vi "WPI_DMARead.vi"(8 "error in (no error)":errorcluster, 9 "Timeout":dbl=5.0, 10 "SamplesToRead":u32=1, 11 "DMARef":T1) -> (0 "error out":errorcluster, 1 "Overrun":bool, 2 "Data":string, 3 "DMARef":T1, 4 "Samples Remaining":u32, 5 "Timed Out":bool)   [LabVIEW 2017]
doc: "Copies and returns the data out of the host buffer.\n\nThis software is licensed. Open the labview\\readme\\WPI Robotics Library Open Source License.txt file for more information."
uses:
  <vilib>/Rock Robotics/WPI/DMA/WPI_DMARef.ctl
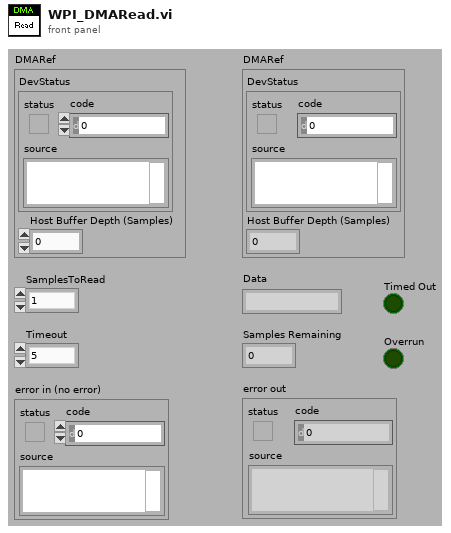
[diagram p1: front panel]
types:
  T1 = typedef "WPI_DMARef.ctl" = cluster{"DevStatus":errorcluster, "Host Buffer Depth (Samples)":u32}
  T2 = typedef "FPGA_DMADevRef.ctl" = cluster{"DevStatus":errorcluster}
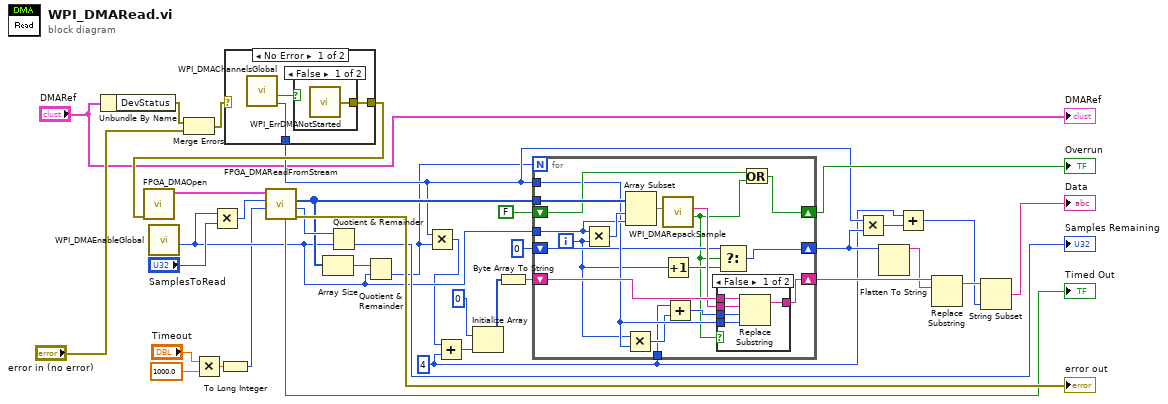
[diagram p0: block diagram]
diagram:
  w6 = u32 4 ("y")
  n1 = Unbundle By Name("DMARef") -> ("DevStatus"=w4:errorcluster)
  n2 = call <vilib>:"WPI_DMAEnableGlobal.vi"() -> ("WordsPerSample"=w21:u16)  [unwired: 2 in, 9 out]
  n3 = Merge Errors(w4, "error in (no error)") -> (w3:errorcluster)
  n4 = Multiply(x="Timeout", y=1000.0) -> (x*y=w29:dbl)
  n5 = Multiply(x=w21, y="SamplesToRead") -> (x*y=w27:u32)
  n6 = To Long Integer(number=w29) -> (32bit integer=w5:i32)
  n7 = case shown="No Error" w3 {
    selector: w3 -> [_ w42]
    tunnel: [w39 w42] -> w32
    tunnel: [w38 _] -> w14
    frame No Error {
      n8 = call <vilib>:"WPI_DMAChannelsGlobal.vi"() -> ("Packed Bytes Per Sample"=w38:i32, "Started"=w40:bool)  [unwired: 4 in, 6 out]
      n9 = case shown="False" w40 {
        tunnel: [w41 _] -> w39
        frame False {
          n10 = call <vilib>:"WPI_ErrDMANotStarted.vi"() -> ("error out"=w41:errorcluster)
        }
        frame True {
        }
      }
    }
    frame Error {
    }
  }
  n11 = call <vilib>:"FPGA_DMAOpen.vi"("error in (no error)"=w32) -> ("DMADevRef"=w28:T2)  [unwired: 10 out]
  n12 = call <vilib>:"FPGA_DMAReadFromStream.vi"("Timeout (ms)"=w5, "NumberOfElements"=w27, "DMADevRef In"=w28) -> ("error out"=→"error out":errorcluster, "Elements Remaining"=w25:u32, "Data"=w23:u32[], "Timed Out"=→"Timed Out":bool)  [unwired: 1 in, 4 out]
  n13 = Array Size(array=w23) -> (size(s)=w24:i32)
  n14 = Quotient & Remainder(x=w25, y=w21) -> (floor(x/y)=→"Samples Remaining":u32)  [unwired: 1 out]
  n15 = Quotient & Remainder(x=w24, y=w21) -> (floor(x/y)=w13:i32)  [unwired: 1 out]
  n16 = Multiply(x=w14, y=w13) -> (x*y=w12:i32)
  n17 = Add(x=w12, y=w6) -> (x+y=w11:u32)
  n18 = Initialize Array(u8 0, w11) -> (w9:u8[])
  n19 = Byte Array To String(unsigned byte array=w9) -> (string=w8:string)
  n20 = for {
    N: w13 -> [_]
    tunnel: w23 -> [w60]
    tunnel: w14 -> [w50]
    shift-right: [w56] -> w34
    shift-left: FALSE -> [w55]
    shift-right: [w54] -> w7
    shift-left: 0 -> [w46]
    tunnel: w21 -> [w57]
    shift-right: [w53] -> w19
    shift-left: w8 -> [w52]
    tunnel: w6 -> [w47]
    i -> [w44]
    n21 = Multiply(x=w57, y=w44) -> (x*y=w58:i32)
    n22 = Multiply(x=w44, y=w50) -> (x*y=w49:i32)
    n23 = Array Subset(array=w60, index=w58, length=w57) -> (w59:u32[])
    n24 = call <vilib>:"WPI_DMARepackSample.vi"("Data"=w59) -> ("Overun"=w43:bool, "String Out"=w51:string)  [unwired: 9 out]
    n25 = Increment(x=w44) -> (x+1=w45:i32)
    n26 = Add(x=w47, y=w49) -> (x+y=w48:u32)
    n27 = case shown="False" w43 {
      tunnel: [w65 w66] -> w53
      tunnel: w52 -> [w64 w66]
      tunnel: w51 -> [w63 _]
      tunnel: w50 -> [w62 _]
      tunnel: w48 -> [w61 _]
      frame False {
        n28 = Replace Substring(2:w62, 3:w61, 4:w63, 5:w64) -> (1:w65:string)  [unwired: 1 out]
      }
      frame True {
      }
    }
    n29 = Select(t=w46, s=w43, f=w45) -> (s? t:f=w54:i32)
    n30 = Or(x=w55, y=w43) -> (x .or. y?=w56:bool)
  }
  "Overrun" <- w34
  n31 = Multiply(x=w14, y=w7) -> (x*y=w16:i32)
  n32 = Flatten To String(anything=w7) -> (data string=w18:string)  [unwired: 1 in, 4 out]
  n33 = Add(x=w6, y=w16) -> (x+y=w15:u32)
  n34 = Replace Substring(4:w18, 5:w19) -> (1:w17:string)  [unwired: 3 out]
  n35 = String Subset(string=w17, length (rest)=w15) -> (substring=→"Data":string)  [unwired: 1 out]
  "DMARef" <- "DMARef"
